vi "LBCB Number 2 Source.vi"(6 "Combined":bool, 10 "LBCB Number":T2) -> (2 "Dataset Source":T1)   [LabVIEW 2013]
uses:
  Data Access Objects/Metadata/LBCB Number.ctl
  Dataset Source.ctl
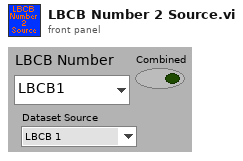
[diagram p1: front panel]
types:
  T1 = typedef "Dataset Source.ctl" = enum16{"LBCB 1", "LBCB 2", "Combined", "External Sensors"}
  T2 = typedef "LBCB Number.ctl" = enum16{"LBCB1", "LBCB2"}
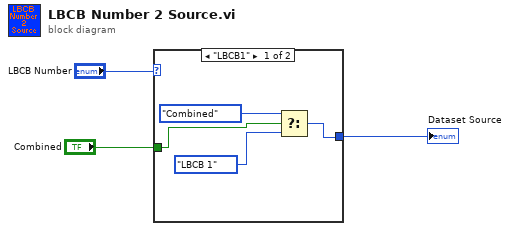
[diagram p0: block diagram]
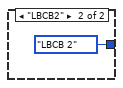
[diagram p2: hidden frame]
diagram:
  n1 = case shown="\"LBCB1\"" "LBCB Number" {
    tunnel: [w6 Dataset_Source."LBCB 2" ("Dataset Source")] -> w2
    tunnel: "Combined" -> [w4 _]
    frame "LBCB1" {
      n2 = Select(t=Dataset_Source."Combined" ("Dataset Source"), s=w4, f=Dataset_Source."LBCB 1") -> (s? t:f=w6:T1)
    }
    frame "LBCB2" {
    }
  }
  "Dataset Source" <- w2
